vi "Agilent 2000 3000_SavingDataCSV_1.vi"() -> ()   [LabVIEW 2016]
doc: "This example shows how to use autosetup and acquire a waveform on a single channel."
uses:
  <vilib>/Waveform/WDTOps.llb/WDT Number of Waveform Samples DBL.vi
  <vilib>/Waveform/WDTOps.llb/WDT Append Waveforms DBL.vi
  <vilib>/Waveform/WDTOps.llb/WDT Waveform Duration DBL.vi
  <vilib>/Waveform/WDTFileIO.llb/Export Waveform To Spreadsheet File.vi
  <instrlib>/Agilent 2000 3000 X-Series/Agilent 2000 3000 X-Series.lvlib
panel:
  out "HardwareAntwort":string
  out "Error_out":errorcluster
  in  "Error_in":errorcluster
  out "number of samples":i32=5000
  out "Y":dbl[](array[numeric])
  out "dt":dbl
  out "t0":timestamp
  in  "Auto Scale Source (0: Channel 1) 3":i32(ring) items=["Channel 1"=0, "Channel 2"=1, "Channel 3"=2, "Channel 4"=3, "Digital Bus Low"=9, "Digital Bus High"=10]
  in  "stop":bool
  in  "Auto Scale Source (0: Channel 1)":i32(ring) items=["Channel 1"=0, "Channel 2"=1, "Channel 3"=2, "Channel 4"=3, "Digital Bus Low"=9, "Digital Bus High"=10]
  in  "Maximum Time (10000 ms)":u32=10000
  out "Waveform Data":waveform(dbl)(graph)
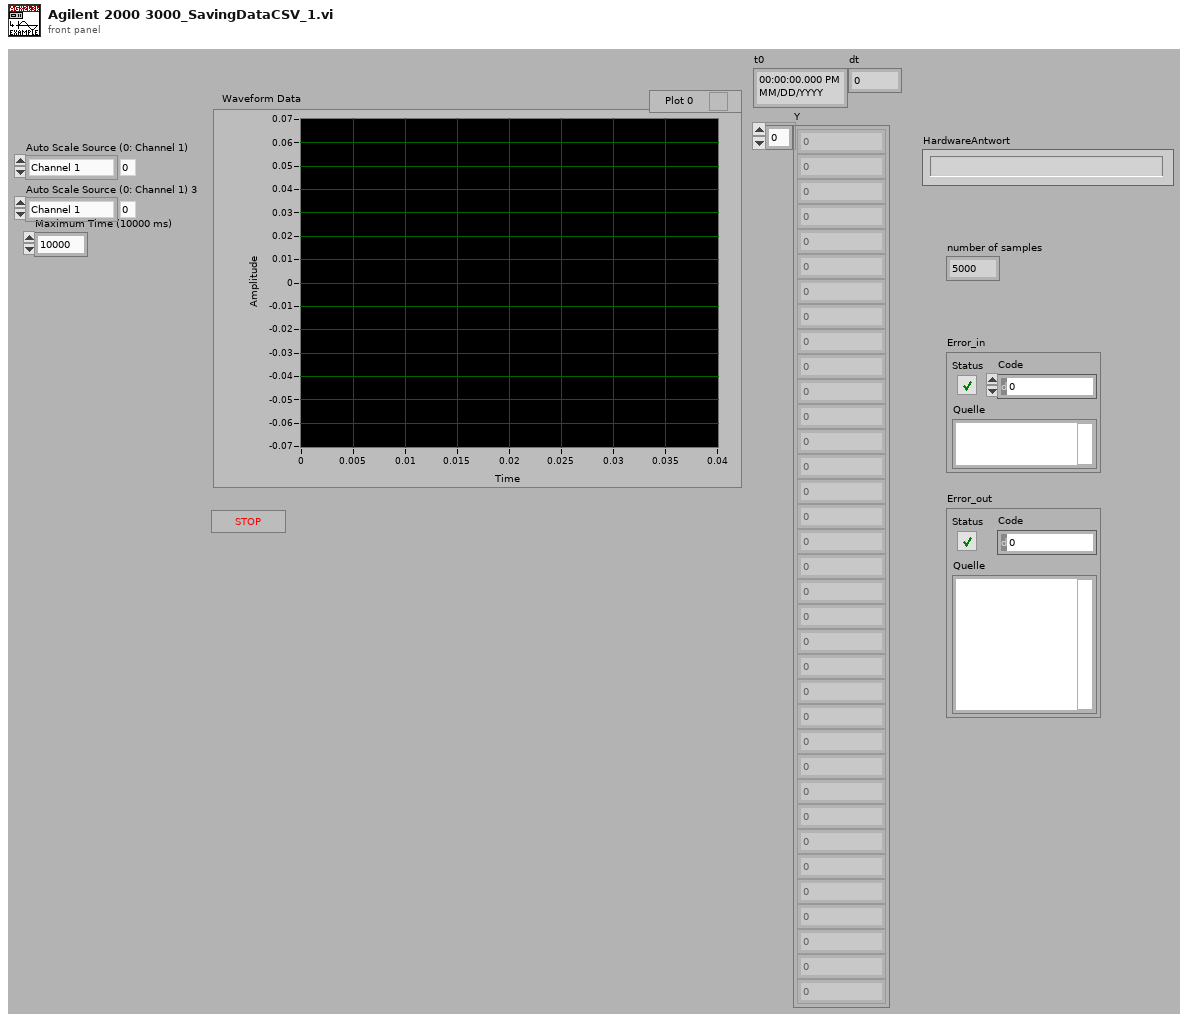
[diagram p1: front panel]
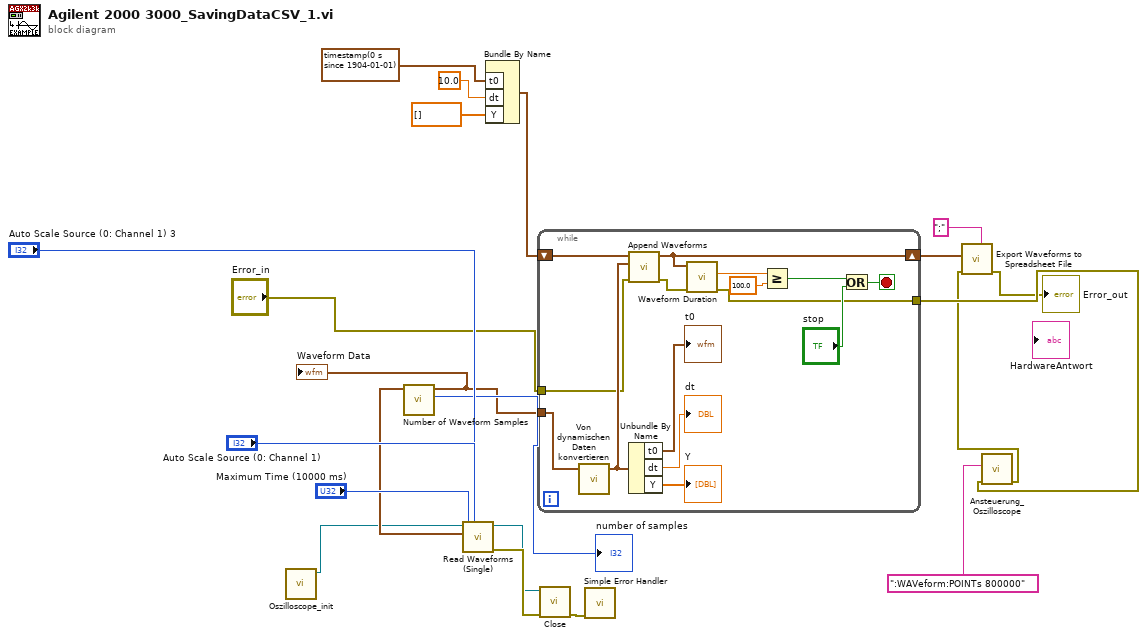
[diagram p0: block diagram]
diagram:
  n1 = call "Oszilloscope_init.vi"() -> ("VISA resource name out"=w5:refnum<visa-resource-name>)  [unwired: 10 in, 1 out]
  n2 = call <instrlib>:"Read Waveforms (Single).vi"("Bind Source Channel (2: None)"="Auto Scale Source (0: Channel 1) 3", "Timeout (10000 ms)"="Maximum Time (10000 ms)", "Source Channel (0: Channel 1)"="Auto Scale Source (0: Channel 1)", "VISA resource name"=w5) -> ("error out"=w20:errorcluster, "Waveform Data"=w6:waveform(dbl), "VISA resource name out"=w19:refnum<visa-resource-name>)  [unwired: 1 in, 4 out]
  n3 = call-poly <vilib>:"Number of Waveform Samples.vi"("waveform in"=w6) -> ("number of samples"=→"number of samples":i32, "waveform out"=w8:waveform(dbl))  [unwired: 8 in, 1 out]
  "Waveform Data" <- w8
  n4 = Bundle By Name("t0"=timestamp(0 s since 1904-01-01), "dt"=10.0, "Y"=dbl[] []) -> (w15:waveform(dbl))  [unwired: 1 in]
  n5 = while {
    shift-right: [w31] -> w10
    shift-left: w15 -> [w33]
    tunnel: w8 -> [w22]
    tunnel: "Error_in" -> [w23]
    tunnel: [w24] -> w3
    stop <- w26 stop-if-true
    n6 = call "Von dynamischen Daten konvertieren"("Dynamic Data Type"=w22) -> ("Waveform"=w32:waveform(dbl))  [unwired: 3 in]
    n7 = call-poly <vilib>:"Append Waveforms.vi"("error in (no error)"=w23, "waveform B"=w32, "waveform A"=w33) -> ("error out"=w25:errorcluster, "waveform out"=w31:waveform(dbl))  [unwired: 7 in]
    n8 = Unbundle By Name(w32) -> ("t0"=→"t0":timestamp, "dt"=→"dt":dbl, "Y"=→"Y":dbl[])
    n9 = call-poly <vilib>:"Waveform Duration.vi"("error in (no error)"=w25, "waveform in"=w31) -> ("error out"=w24:errorcluster, "duration"=w30:dbl)  [unwired: 7 in, 1 out]
    n10 = Greater Or Equal?(x=w30, y=100.0) -> (x >= y?=w27:bool)
    n11 = Or(x=w27, y="stop") -> (x .or. y?=w26:bool)
  }
  n12 = call <instrlib>:"Close.vi"("error in (no error)"=w20, "VISA resource name"=w19) -> ("error out"=w21:errorcluster)  [unwired: 9 out]
  n13 = call <vilib>:"Simple Error Handler.vi"("error in (no error)"=w21) -> ()  [unwired: 1 in, 8 out]
  n14 = call "Ansteuerung_Oszilloscope.vi"("Error_in"=w3, "Eingangs-String"=":WAVeform:POINTs 800000" ("format string")) -> ("Error_out"=w1:errorcluster)  [unwired: 7 in, 2 out]
  n15 = call-poly <vilib>:"Export Waveforms to Spreadsheet File.vi"("delimiter (Tab)"=";", "error in (no error)"=w1, "waveform"=w10) -> ("error out"=→"Error_out":errorcluster)  [unwired: 7 in, 1 out]
